vi "Get Action Names.vi"() -> (0 "Names":T1[](array[typedef]))   [LabVIEW 2021]
uses:
  Sub Controls/Instrument Info.ctl
  New NML Data Acq/Sub Controls/Instrument Actions.ctl
  New NML Data Acq/Sub Controls/Instrument Ref.ctl
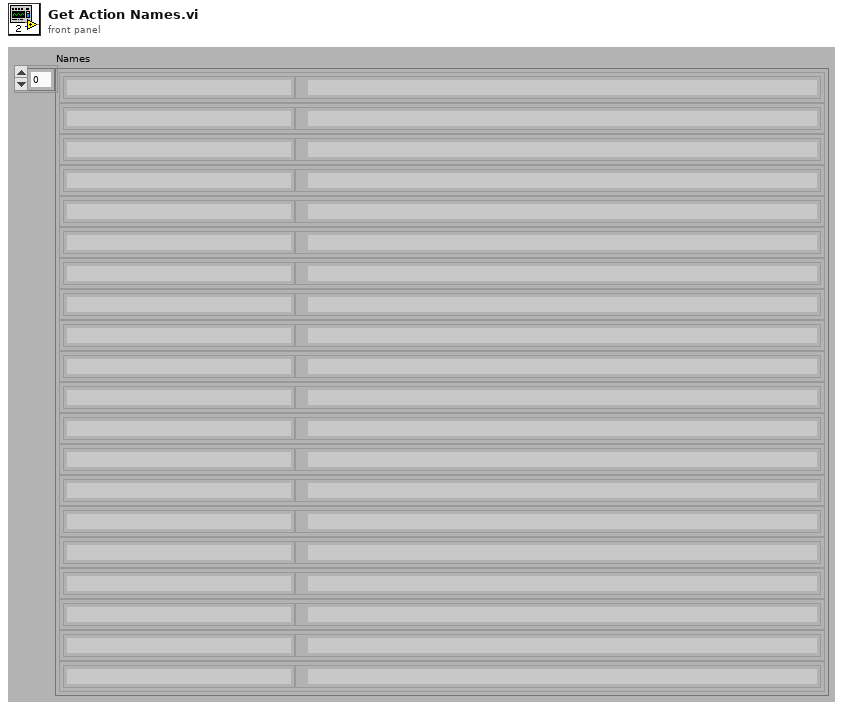
[diagram p1: front panel]
types:
  T1 = typedef "Instrument Info.ctl" = cluster{"Name":string, "path":path}
  T2 = typedef "Instrument Actions.ctl" = enum16{"Scan", "Identify", "New", "Configure", "Initialize", "Test", "Read", "Close"}
  T3 = typedef "Instrument Ref.ctl" = refnum<vi>
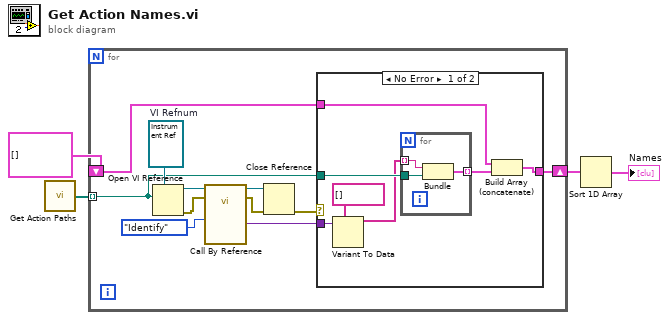
[diagram p0: block diagram]
diagram:
  n1 = call "Get Action Paths.vi"() -> ("paths"=w4:path[])  [unwired: 1 in]
  n2 = for {
    tunnel: w4 -> [w5] mode=indexing
    shift-right: [w12] -> w2
    shift-left: cluster{string, "appended path":path}[] [] -> [w11]
    w6 = T3 refnum  # VI Refnum
    n3 = Open VI Reference(type specifier VI Refnum (for type only)=w6, vi path=w5) -> (vi reference=w15:T3, error out=w14:errorcluster)  [unwired: 4 in]
    n4 = call-by-ref "?"(reference=w15, error in=w14, "Action"=Instrument_Actions."Identify") -> (reference out=w8:T3, error out=w10:errorcluster, "Output"=w13:variant)  [unwired: 5 in, 1 out]
    n5 = Close Reference(reference=w8, error in (no error)=w10) -> (error out=w9:errorcluster)
    n6 = case shown="No Error" w9 {
      tunnel: w13 -> [w22 _]
      tunnel: w5 -> [w21 _]
      tunnel: [w20 w26] -> w12
      tunnel: w11 -> [w18 w26]
      frame No Error {
        n7 = Variant To Data(type=string[] [], Variant=w22) -> (data=w17:string[])  [unwired: 1 in, 1 out]
        n8 = for {
          tunnel: w21 -> [w23]
          tunnel: [w25] -> w19 mode=indexing
          tunnel: w17 -> [w24] mode=indexing
          n9 = Bundle(w24, "appended path"=w23) -> (w25:cluster{string, "appended path":path})  [unwired: 1 in]
        }
        n10 = Build Array (concatenate)(w18, w19) -> (w20:cluster{string, "appended path":path}[])
      }
      frame Error {
      }
    }
  }
  n11 = Sort 1D Array(array=w2) -> (sorted array=→"Names":cluster{string, "appended path":path}[])
